vi "SpreadsheetRead (1).vi"() -> (1 "XY Graph":cluster{"all rows":dbl[], "all rows":dbl[]}(graph))   [LabVIEW 2015]
uses:
  <vilib>/Utility/file.llb/Read Delimited Spreadsheet (DBL).vi
panel:
  out "Output Cluster":cluster{"Column 0":dbl[], "Column 1":dbl[]}
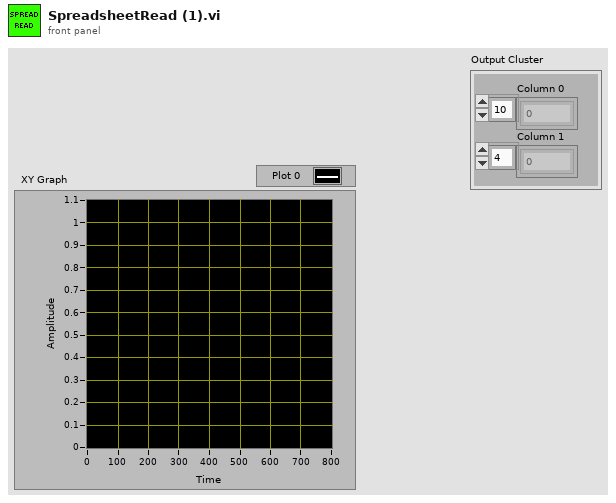
[diagram p1: front panel]
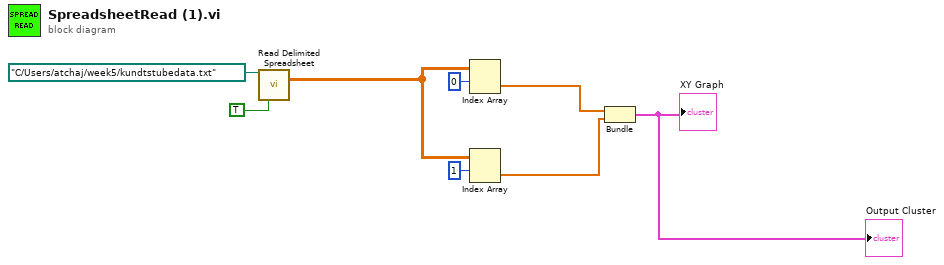
[diagram p0: block diagram]
diagram:
  n1 = call-poly <vilib>:"Read Delimited Spreadsheet.vi"("file path (dialog if empty)"=path "C:/Users/atchaj/week5/kundtstubedata.txt", "transpose? (F)"=TRUE) -> ("all rows"=w6:dbl[][])  [unwired: 8 in, 5 out]
  n2 = Index Array(array=w6, index (row)=0 ("index")) -> (element=w5:dbl[])  [unwired: 1 in]
  n3 = Index Array(array=w6, index (row)=1 ("index")) -> (element=w4:dbl[])  [unwired: 1 in]
  n4 = Bundle("all rows"=w5, "all rows"=w4) -> (→"XY Graph" →"Output Cluster":cluster{"all rows":dbl[], "all rows":dbl[]})  [unwired: 1 in]
